vi "Attendance.vi"() -> ()   [LabVIEW 2017]
panel:
  in  "?":bool
  in  "?":bool
  in  "?":bool
  in  "?":bool
  in  "?":bool
  in  "?":bool
  in  "?":bool
  in  "?":bool
  in  "?":bool
  in  "?":bool
  in  "?":bool
  in  "?":bool
  in  "?":bool
  in  "?":bool
  in  "?":bool
  in  "?":bool
  in  "?":bool
  in  "?":bool
  in  "?":bool
  in  "?":bool
  in  "Operation":u16(ring) items=["Input File as Path", "Input File as Refnum", "Specifying a Format String"]
  out "Read Time":timestamp
  out "Read Boolean":bool
  out "Read String":string
  out "Write Time":timestamp
  in  "Write Boolean":bool
  in  "Write String":string="sample_string"
  in  "Format String":string="Path Value - %s\nString Value - %s\nBoolean Value - %s\nNumeric Value - %d\nTimestamp Value - %T"
  in  "?":bool
  in  "?":bool
  in  "?":bool
  in  "?":bool
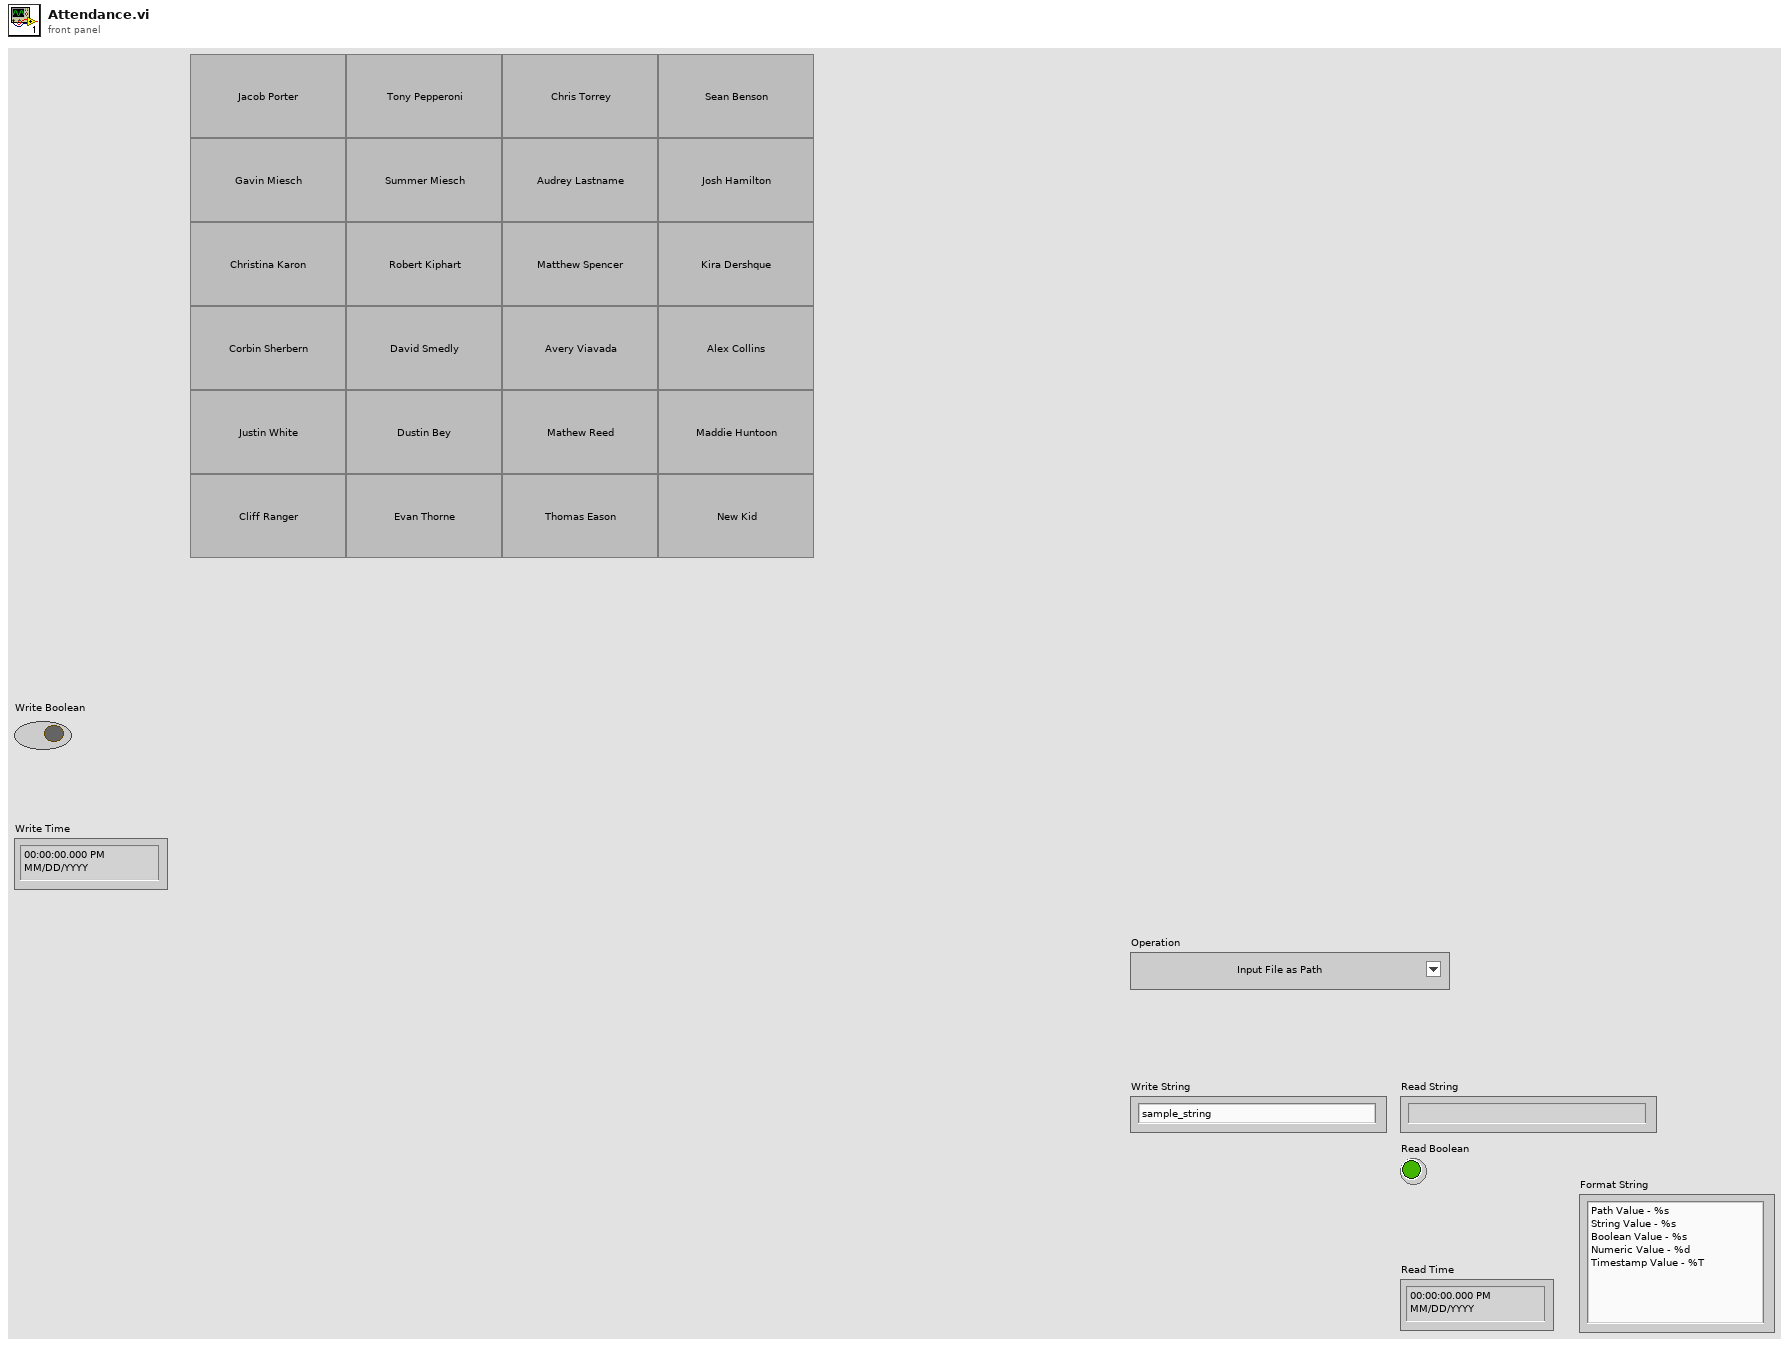
[diagram p1: front panel]
types:
  T1 = enum16{"open", "replace", "create", "open or create", "replace or create", "replace or create with confirmation"}
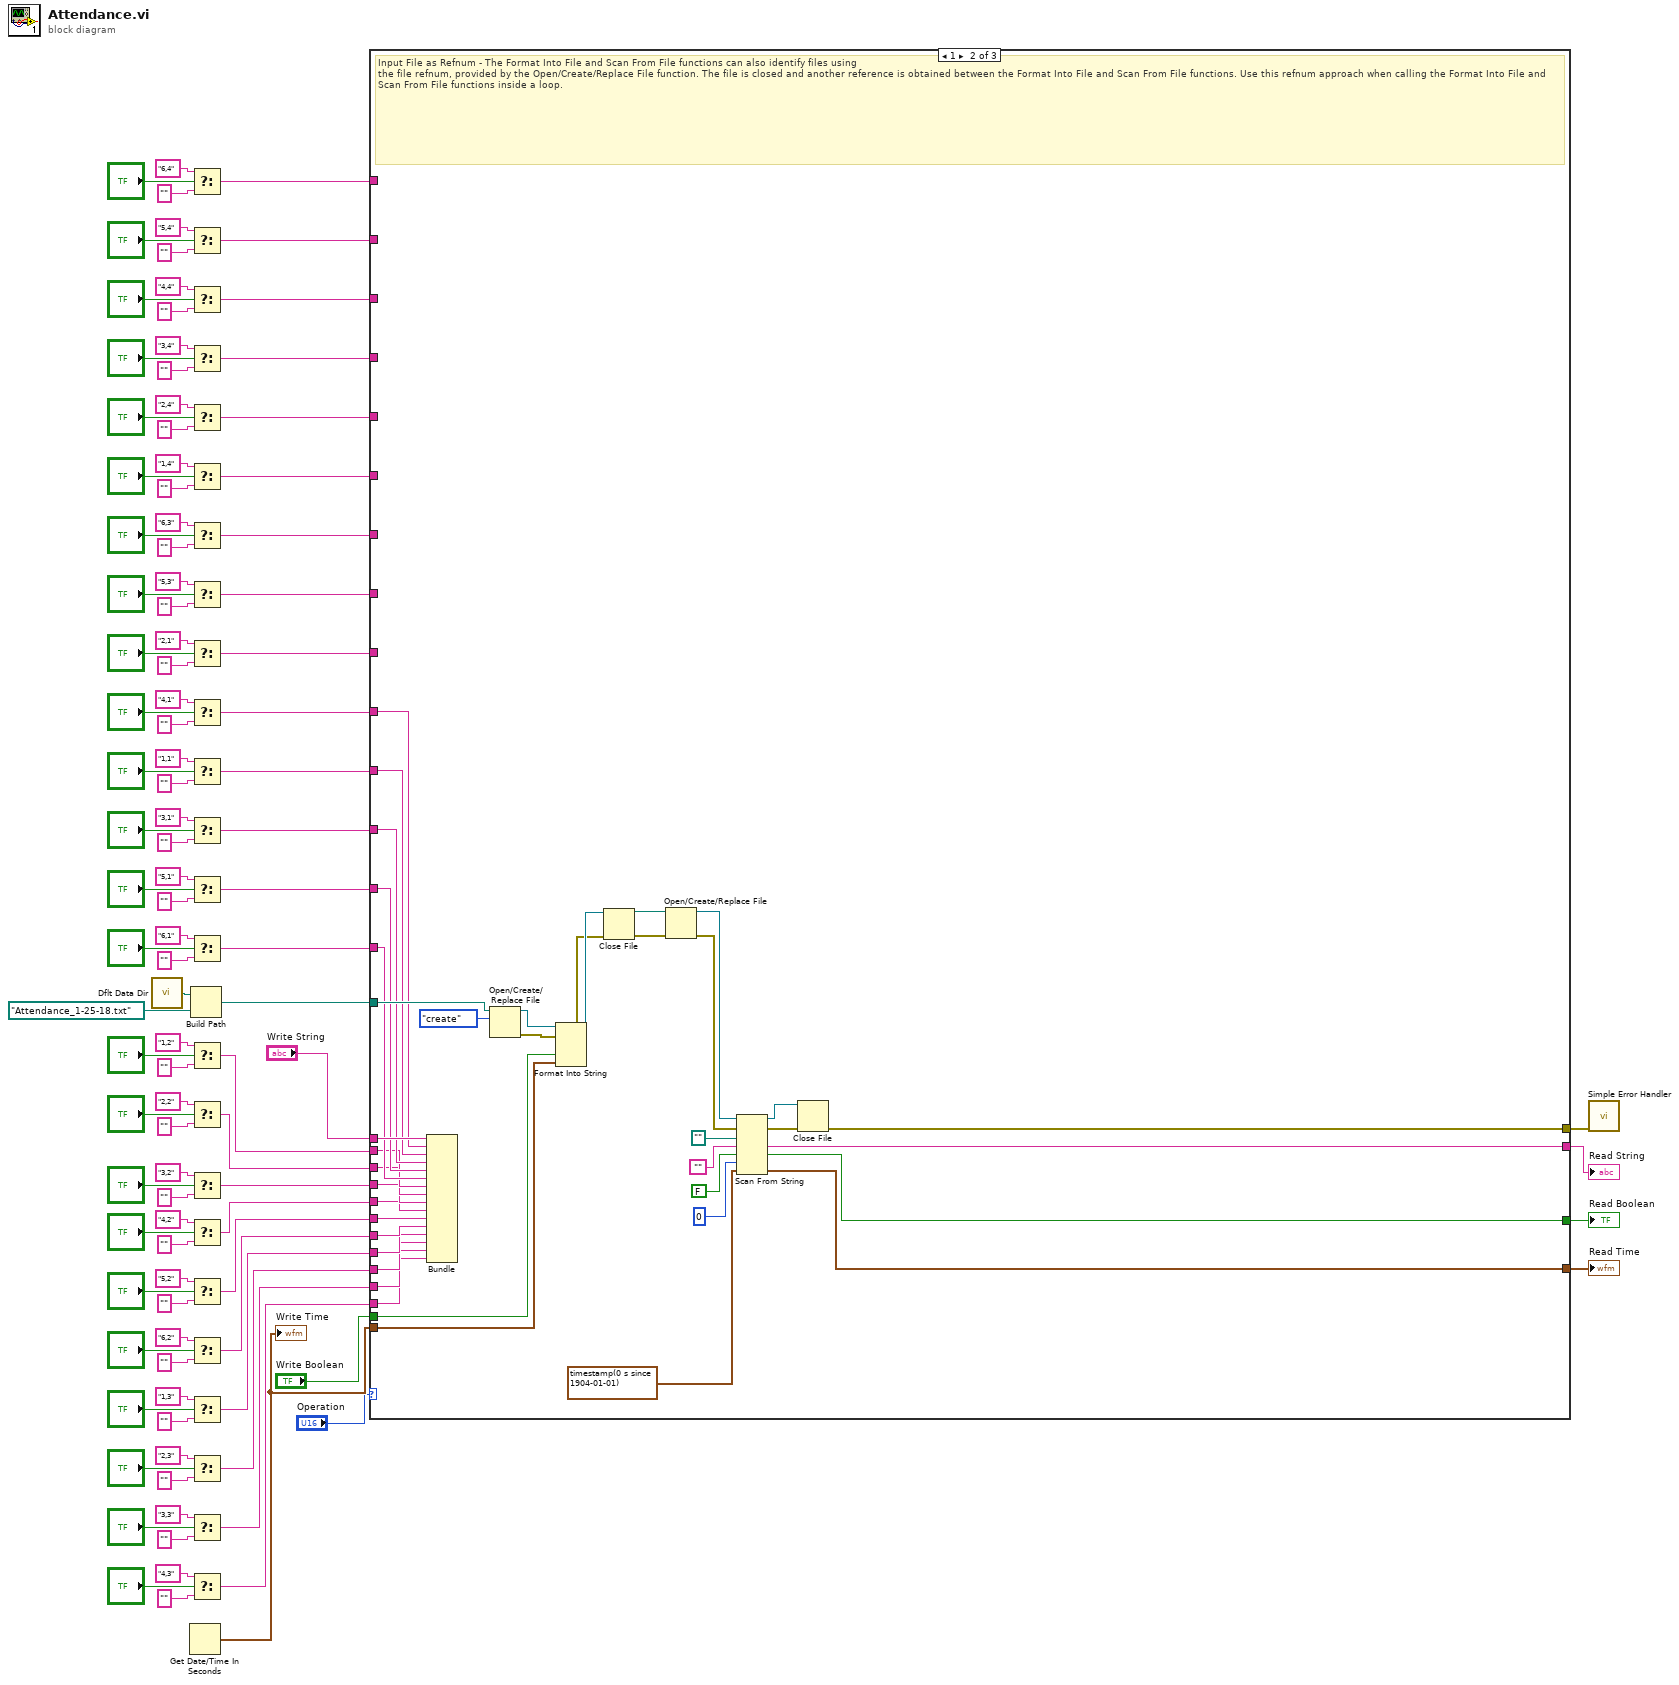
[diagram p0: block diagram]
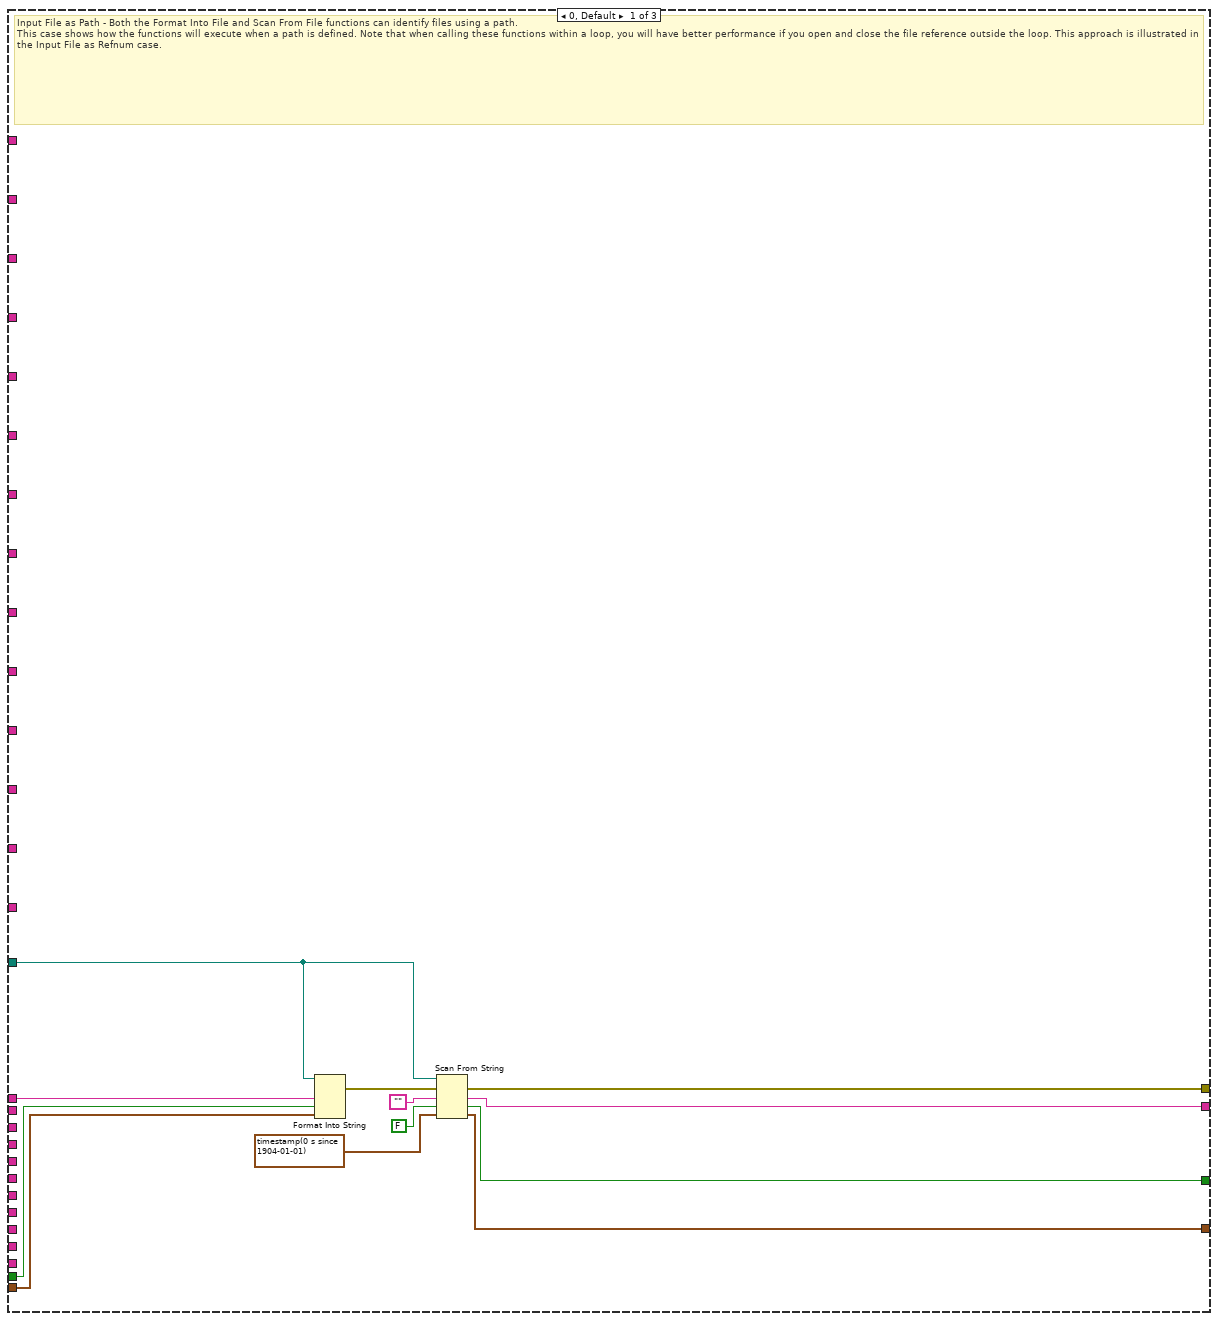
[diagram p2: hidden frame]
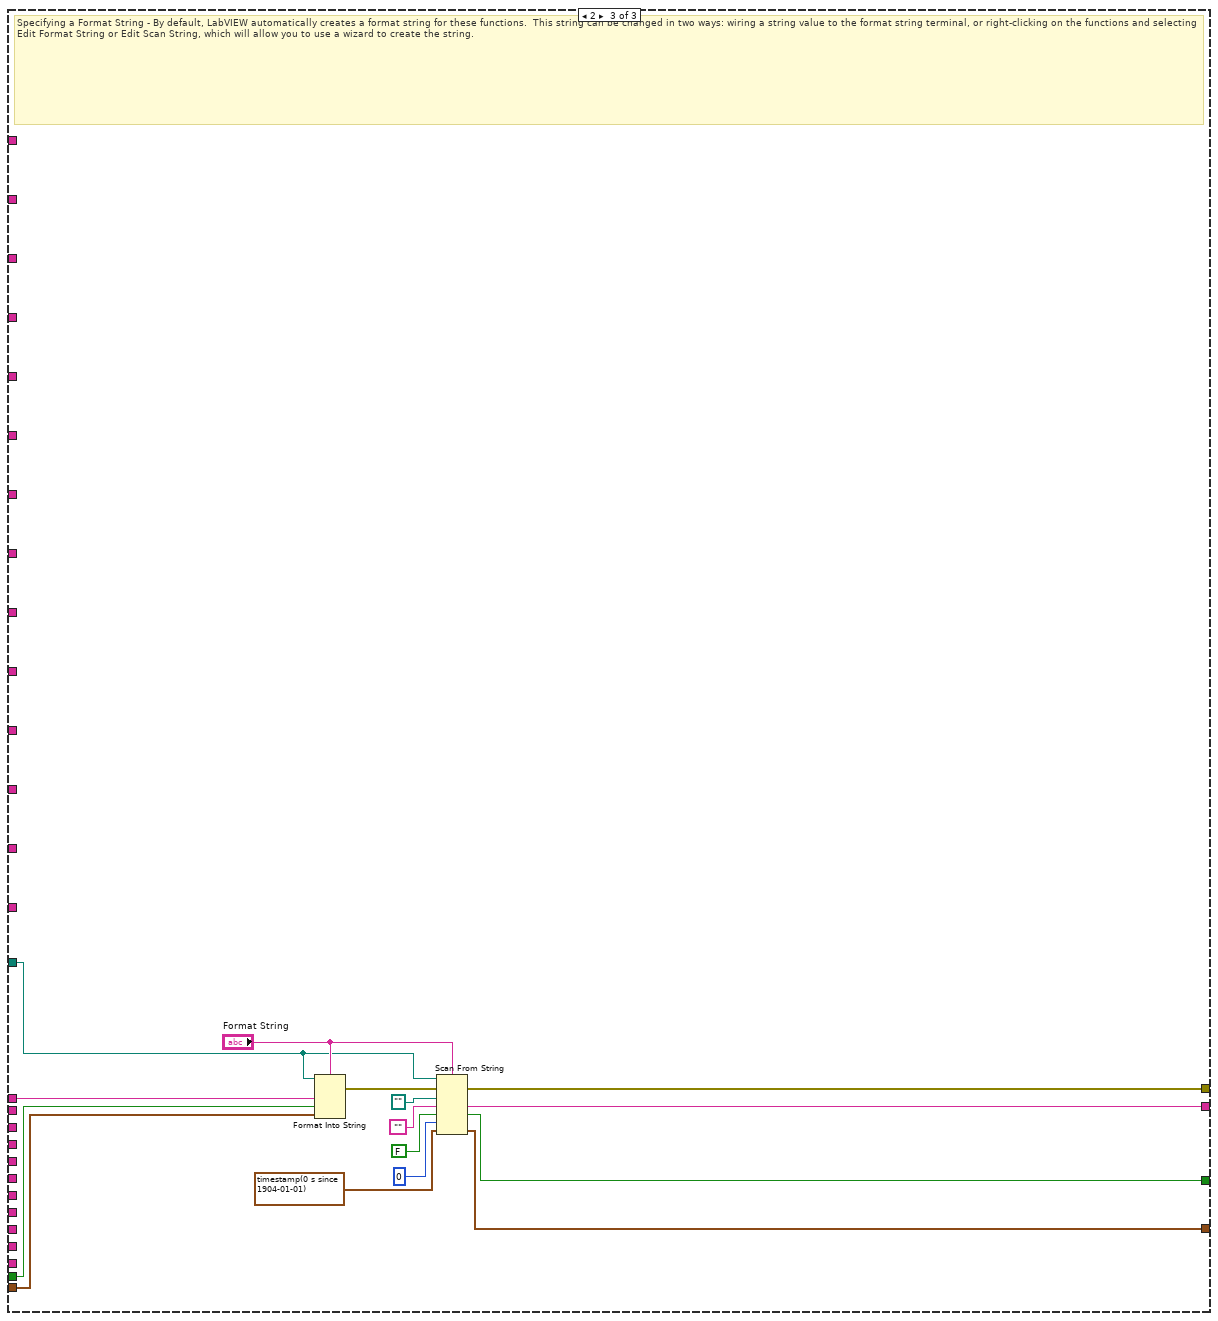
[diagram p3: hidden frame]
diagram:
  n1 = call <vilib>:"Dflt Data Dir.vi"() -> ("App:Default Data Directory"=w91:path)
  n2 = Get Date/Time In Seconds() -> (seconds since 1Jan1904=w97:timestamp)
  "Write Time" <- w97
  n3 = Build Path(base path=w91, name or relative path=path "Attendance_1-25-18.txt" ("default name")) -> (appended path=w89:path)
  n4 = Select(t="6,4", s="?", f="") -> (s? t:f=w1:string)
  n5 = Select(t="5,4", s="?", f="") -> (s? t:f=w5:string)
  n6 = Select(t="4,4", s="?", f="") -> (s? t:f=w6:string)
  n7 = Select(t="3,4", s="?", f="") -> (s? t:f=w7:string)
  n8 = Select(t="2,4", s="?", f="") -> (s? t:f=w8:string)
  n9 = Select(t="1,4", s="?", f="") -> (s? t:f=w9:string)
  n10 = Select(t="6,3", s="?", f="") -> (s? t:f=w43:string)
  n11 = Select(t="5,3", s="?", f="") -> (s? t:f=w44:string)
  n12 = Select(t="2,1", s="?", f="") -> (s? t:f=w87:string)
  n13 = Select(t="4,1", s="?", f="") -> (s? t:f=w85:string)
  n14 = Select(t="1,1", s="?", f="") -> (s? t:f=w88:string)
  n15 = Select(t="3,1", s="?", f="") -> (s? t:f=w86:string)
  n16 = Select(t="5,1", s="?", f="") -> (s? t:f=w76:string)
  n17 = Select(t="6,1", s="?", f="") -> (s? t:f=w75:string)
  n18 = Select(t="1,2", s="?", f="") -> (s? t:f=w74:string)
  n19 = Select(t="2,2", s="?", f="") -> (s? t:f=w73:string)
  n20 = Select(t="3,2", s="?", f="") -> (s? t:f=w52:string)
  n21 = Select(t="4,2", s="?", f="") -> (s? t:f=w51:string)
  n22 = Select(t="5,2", s="?", f="") -> (s? t:f=w50:string)
  n23 = Select(t="6,2", s="?", f="") -> (s? t:f=w49:string)
  n24 = Select(t="1,3", s="?", f="") -> (s? t:f=w48:string)
  n25 = Select(t="2,3", s="?", f="") -> (s? t:f=w47:string)
  n26 = Select(t="3,3", s="?", f="") -> (s? t:f=w46:string)
  n27 = Select(t="4,3", s="?", f="") -> (s? t:f=w45:string)
  n28 = case shown="1" "Operation" {
    tunnel: [w118 w149 w171] -> w90
    tunnel: "Write String" -> [w117 w135 w170]
    tunnel: "Write Boolean" -> [w116 w147 w169]
    tunnel: w97 -> [w113 w146 w168]
    tunnel: [w111 w138 w162] -> w96
    tunnel: [w110 w139 w161] -> w95
    tunnel: [w109 w140 w160] -> w94
    tunnel: w89 -> [w108 w137 w159]
    tunnel: w88 -> [_ w133 _]
    tunnel: w87 -> [_ _ _]
    tunnel: w86 -> [_ w132 _]
    tunnel: w85 -> [_ w134 _]
    tunnel: w76 -> [_ w131 _]
    tunnel: w75 -> [_ w130 _]
    tunnel: w74 -> [_ w129 _]
    tunnel: w73 -> [_ w128 _]
    tunnel: w52 -> [_ w127 _]
    tunnel: w51 -> [_ w126 _]
    tunnel: w50 -> [_ w125 _]
    tunnel: w49 -> [_ w124 _]
    tunnel: w48 -> [_ w123 _]
    tunnel: w47 -> [_ w122 _]
    tunnel: w46 -> [_ w121 _]
    tunnel: w45 -> [_ w120 _]
    tunnel: w44 -> [_ _ _]
    tunnel: w43 -> [_ _ _]
    tunnel: w9 -> [_ _ _]
    tunnel: w8 -> [_ _ _]
    tunnel: w7 -> [_ _ _]
    tunnel: w6 -> [_ _ _]
    tunnel: w5 -> [_ _ _]
    tunnel: w1 -> [_ _ _]
    frame 0, Default {
      # "Input File as Path - Both the Format Into File and Scan From File functions can identify files using a path.  \nThis case shows how the functions will execute when a path is defined. Note that when calling these functions within a loop, you will have better performance if you open and close the file reference outside the loop. This approach is illustrated in the Input File as Refnum case."
      n29 = Format Into String(initial string=w108, w117, w116, w113) -> (error out=w119:errorcluster)  [unwired: 2 in, 1 out]
      n30 = Scan From String(w108, w119, default 1="", default 2=FALSE, default 3=timestamp(0 s since 1904-01-01) ("seconds since 1Jan1904")) -> (w118:errorcluster, output 1=w111:string, output 2=w110:bool, output 3=w109:timestamp)  [unwired: 1 in, 1 out]
    }
    frame 1 {
      # "Input File as Refnum - The Format Into File and Scan From File functions can also identify files using \nthe file refnum, provided by the Open/Create/Replace File function. The file is closed and another reference is obtained between the Format Into File and Scan From File functions. Use this refnum approach when calling the Format Into File and Scan From File functions inside a loop."
      n31 = Bundle("Write String"=w135, w134, w133, w132, w131, w130, w129, w128, w127, w126, w125, w124, w123, w122, w121, w120) -> ()  [unwired: 1 in, 1 out]
      n32 = Open/Create/Replace File(file path (use dialog)=w137, operation (0:open)=T1."create") -> (refnum out=w157:refnum<file>, error out=w151:errorcluster)  [unwired: 1 in, 4 out]
      n33 = Format Into String(initial string=w157, error in=w151, w147, w146) -> (resulting string=w156:refnum<file>, error out=w152:errorcluster)  [unwired: 2 in]
      n34 = Close File(refnum=w156, error in=w152) -> (path=w155:path, error out=w154:errorcluster)
      n35 = Open/Create/Replace File(file path (use dialog)=w155, error in=w154) -> (refnum out=w136:refnum<file>, error out=w148:errorcluster)  [unwired: 5 out]
      n36 = Scan From String(w136, w148, default 1=path "", default 2="", default 3=FALSE, default 4=0, default 5=timestamp(0 s since 1904-01-01) ("seconds since 1Jan1904")) -> (w153:refnum<file>, w150:errorcluster, output 2=w138:string, output 3=w139:bool, output 5=w140:timestamp)  [unwired: 1 in, 2 out]
      n37 = Close File(refnum=w153, error in=w150) -> (error out=w149:errorcluster)  [unwired: 1 out]
    }
    frame 2 {
      # "Specifying a Format String - By default, LabVIEW automatically creates a format string for these functions.  This string can be changed in two ways: wiring a string value to the format string terminal, or right-clicking on the functions and selecting Edit Format String or Edit Scan String, which will allow you to use a wizard to create the string."
      n38 = Format Into String(format string="Format String", initial string=w159, w170, w169, w168) -> (error out=w172:errorcluster)  [unwired: 1 in, 1 out]
      n39 = Scan From String("Format String", w159, w172, default 1=path "", default 2="", default 3=FALSE, default 4=0, default 5=timestamp(0 s since 1904-01-01) ("seconds since 1Jan1904")) -> (w171:errorcluster, output 2=w162:string, output 3=w161:bool, output 5=w160:timestamp)  [unwired: 3 out]
    }
  }
  "Read String" <- w96
  "Read Boolean" <- w95
  "Read Time" <- w94
  n40 = call <vilib>:"Simple Error Handler.vi"("error in (no error)"=w90) -> ()  [unwired: 1 in, 8 out]
